vi "Get Shooter RPM.vi"(9 "Right Shooter Wheel":T1={"DeviceStatus"={"status"=FALSE, "code"=0, "source"=""}, "Type"=enum."PWM", "PWM"={"PWM Channel"=enum."Invalid", "DeadBand"={"Name"="", "maxPositivePwm"=0, "minPositivePwm"=0, "centerPwm"=0, "maxNegativePwm"=0, "minNegativePwm"=0, "angularRange"=0}}, "CAN"={"Device Number"=0, "Control Mode"=enum."Percent VBus", "Semaphore"=refnum, "Max Vout"=12.0, "TalonSRX Control Mode"=enum."Percent VBus"}, "Invert"=FALSE}, 11 "Left Shooter Wheel":T1={"DeviceStatus"={"status"=FALSE, "code"=0, "source"=""}, "Type"=enum."PWM", "PWM"={"PWM Channel"=enum."Invalid", "DeadBand"={"Name"="", "maxPositivePwm"=0, "minPositivePwm"=0, "centerPwm"=0, "maxNegativePwm"=0, "minNegativePwm"=0, "angularRange"=0}}, "CAN"={"Device Number"=0, "Control Mode"=enum."Percent VBus", "Semaphore"=refnum, "Max Vout"=12.0, "TalonSRX Control Mode"=enum."Percent VBus"}, "Invert"=FALSE}) -> (1 "Average RPM":dbl, 2 "Right RPM":dbl, 3 "Left RPM":dbl)   [LabVIEW 2015]
uses:
  <vilib>/Rock Robotics/WPI/MotorControl/WPI_MotorControlDeviceRef.ctl
  <vilib>/Rock Robotics/WPI/MotorControl/WPI_MotorControlType.ctl
  <vilib>/Rock Robotics/SystemInterfaces/DIO/FPGA_DIOPWMChannel.ctl
  <vilib>/Rock Robotics/WPI/PWM/WPI_PWMDeadband.ctl
  <vilib>/Rock Robotics/WPI/CAN/Jaguar/SubVIs/WPI_CANJaguar_ControlMode.ctl
  <vilib>/Rock Robotics/WPI/CAN/TalonSRX/WPI_CANTalonSRX_APIControlMode.ctl
  <vilib>/Rock Robotics/WPI/CAN/TalonSRX/WPI_CANTalonSRX_APIFeedbackSelect.ctl
  Robot Global Data.vi
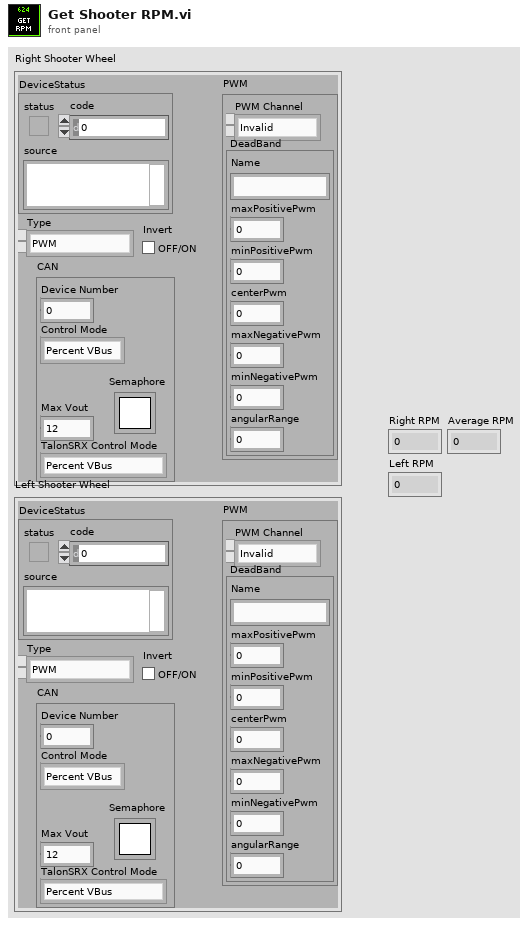
[diagram p1: front panel]
types:
  T1 = typedef "WPI_MotorControlDeviceRef.ctl" = cluster{"DeviceStatus":errorcluster, "Type":T2, "PWM":cluster{"PWM Channel":T3, "DeadBand":T4}, "CAN":cluster{"Device Number":u8, "Control Mode":T5, "Semaphore":T6, "Max Vout":dbl, "TalonSRX Control Mode":T7}, "Invert":bool}
  T2 = typedef "WPI_MotorControlType.ctl" = enum16{"PWM", "CAN", "CANTalonSRX"}
  T3 = typedef "FPGA_DIOPWMChannel.ctl" = enum8{"PWM 0", "PWM 1", "PWM 2", "PWM 3", "PWM 4", "PWM 5", "PWM 6", "PWM 7", "PWM 8", "PWM 9", "PWM MXP 0", "PWM MXP 1", "PWM MXP 2", "PWM MXP 3", "PWM MXP 4", "PWM MXP 5", "PWM MXP 6", "PWM MXP 7", "PWM MXP 8", "PWM MXP 9", "Invalid"}
  T4 = typedef "WPI_PWMDeadband.ctl" = cluster{"Name":string, "maxPositivePwm":i32, "minPositivePwm":i32, "centerPwm":i32, "maxNegativePwm":i32, "minNegativePwm":i32, "angularRange":u16}
  T5 = typedef "WPI_CANJaguar_ControlMode.ctl" = enum8{"Percent VBus", "Current", "Speed", "Position", "Voltage"}
  T6 = typedef "Semaphore RefNum" = refnum<k1>
  T7 = typedef "WPI_CANTalonSRX_APIControlMode.ctl" = enum8{"Percent VBus", "Speed", "Position", "Slave", "Unchanged / Invalid", "Voltage Compensation", "Current", "Motion Profile"}
  T8 = typedef "WPI_CANTalonSRX_APIFeedbackSelect.ctl" = enum16{"Digital Quadrature Encoder", "Analog Potentiometer", "Analog Encoder", "Count on Quad-A (Rising-Edge)", "Count on Quad-A (Falling-Edge)", "CTR Magnetic Enc (Absolute)", "CTR Magnetic Enc (Relative)", "Pulse Width"}
  T9 = typedef "Dashboard Control Data.ctl" = cluster{"Shooter Presets":T10, "Encoder Control":T12, "Steer PID output":cluster{"output high":dbl, "output low":dbl}, " Steer PID gains":cluster{"proportional gain (Kc)":dbl, "integral time (Ti, min)":dbl, "derivative time (Td, min)":dbl}, "Drivetrain Settings":T13, "Vision Packet":T14, "Dashboard Drivetrain Command":T15, "Info/Command Cluster":T17, "Ball Vision Packet":T18, "Intake Presets":T20, "Intake Encoder Control":T22, "Climb Presets":T23, "Ultrasonic Limit":dbl, "Roll Limit":dbl, "Pitch Limit":dbl, "Goal Output Range":cluster{"output high":dbl, "output low":dbl}}
  T10 = typedef "Shooter Presets.ctl" = cluster{"Batter Shot":T11, "Deep Middle Shot":T11, "Manual Shot":T11, "Left Ticks Per Rotation":dbl, "Right Ticks Per Rotation":dbl, "Low Bar Shot":T11, "Shooter RPM Tolerance":dbl, "IIR Filter Power":dbl, "Trigger Power":dbl, "Fire from Load Delay":i32, "Angle Pot M":dbl, "Angle Pot B":dbl, "Shooter Length":dbl, "String Pot Dist":dbl, "Angle PID gains":cluster{"proportional gain (Kc)":dbl, "integral time (Ti, min)":dbl, "derivative time (Td, min)":dbl}, "Angle Motor Output":cluster{"output high":dbl, "output low":dbl}, "Shooter Angle Tolerance":dbl, "Vision Shoot x^2":dbl, "Vision Shoot x":dbl, "Dist from Axis Cam to Pivot":dbl, "High Goal Center Height":dbl, "Feed Forward Max Accel":dbl, "Feed Forward Kv":dbl, "Backwards Trigger":dbl, "Shot Finish Delay (ms)":dbl, "Angle Max Current":dbl, "Angle Current Trip Time":dbl, "Shooter Intake Angle":dbl, "Vision Shoot c":dbl, "Reset?":bool, "Servo Release Delay":dbl, "Servo Idle Angle":i32, "Servo Hold Angle":i32, "Angle Pot x^2":dbl, "Angle Pot x":dbl, "Angle Pot c":dbl, "Ignore Angle?":bool}
  T11 = typedef "Shot Presets.ctl" = cluster{"Left Wheel RPM":dbl, "Right Wheel RPM":dbl, "Angle":dbl}
  T12 = typedef "Encoder Control.ctl" = cluster{"Right Tick Constant":dbl, "Left Tick Constant":dbl, "Reset?":bool, "Y Dist":cluster{"PID gains":cluster{"proportional gain (Kc)":dbl, "integral time (Ti, min)":dbl, "derivative time (Td, min)":dbl}}, "Y Stop Thresh":dbl, "Y Stop Speed":dbl}
  T13 = typedef "Drivetrain Settings.ctl" = cluster{"Gyro Tolerance":dbl, "Throttle Ramp (ms)":dbl, "Angular rate compensation":bool, "Throttle to Rate Scale":dbl, "Rate compensation gain":dbl, "Kv":dbl, "Ka":dbl, "Feed Forward P":dbl, "Feed Forward D":dbl, "Goal Vision PID gains":cluster{"proportional gain (Kc)":dbl, "integral time (Ti, min)":dbl, "derivative time (Td, min)":dbl}, "Goal Detection Window":dbl}
  T14 = typedef "Goal Vision Packet.ctl" = cluster{"Distance":dbl, "Center X":dbl, "Center Y":dbl, "Found Target?":bool}
  T15 = typedef "Dashboard Drivetrain Command.ctl" = cluster{"Drivetrain Vision":T16}
  T16 = typedef "Drivetrain Vision.ctl" = cluster{"Goal Window":dbl, "Ball Window":dbl}
  T17 = typedef "Ball Tracking Command Cluster.ctl" = cluster{"Distance to Ball":dbl, "Desired Angle":dbl, "Command":enum16{"Turn to Ball", "Turn to Angle", "Get Distance"}, "Pixels from Center":dbl}
  T18 = typedef "Ball Vision Packet.ctl" = cluster{"Ball Detected?":bool, "Distance to Ball":dbl, "Desired Angle":dbl, "Pixels from Center":dbl, "Tracking mode":T19}
  T19 = typedef "Tracking Mode.ctl" = enum16{"Turn to Ball", "Turn to Angle"}
  T20 = typedef "Intake Presets.ctl" = cluster{"Intake Speed":dbl, "Outake Speed":dbl, "Low Height":dbl, "Half Height":dbl, "Full Height":dbl, "Angle Speed":dbl, "Fast Angle":dbl, "Encoder Scale":dbl, "Load Height":dbl, "Output Range":T21, "Rotation Power Max/Min":dbl, "MaxCurrent":dbl, "Intake Trip Time":dbl, "Idle Height":dbl, "Max Height":dbl, "Reset Encoders?":bool, "PID gains":cluster{"proportional gain (Kc)":dbl, "integral time (Ti, min)":dbl, "derivative time (Td, min)":dbl}}
  T21 = typedef "Drivetrain Output Range.ctl" = cluster{"output high":dbl, "output low":dbl}
  T22 = typedef "IntakeEcoderControl.ctl" = cluster{"Arm Tick Constant":dbl, "Reset?":bool, "Y Dist":cluster{"PID gains":cluster{"proportional gain (Kc)":dbl, "integral time (Ti, min)":dbl, "derivative time (Td, min)":dbl}}, "Y Stop Thresh":dbl, "Y Stop Speed":dbl}
  T23 = typedef "Climb Presets.ctl" = cluster{"Pull Power":dbl, "Unpin Power":dbl, "Time to Hold":dbl}
  T24 = typedef "WPI_CANTalonSRX_GlobalStatus.ctl" = cluster{"Applied Throttle":dbl, "Module Enabled":bool, "CAN Error":errorcluster, "Closed Loop Error":dbl, "Forward Limit Switch Closed":bool, "Reverse Limit Switch Closed":bool, "Sensor Position":dbl, "Sensor Velocity":dbl, "Current":dbl, "Sticky Fault - Over Temp":bool, "Sticky Fault - Under Voltage":bool, "Sticky Fault - Forward Limit":bool, "Sticky Fault - Reverse Limit":bool, "Sticky Fault - Forward Soft Limit":bool, "Sticky Fault - Reverse Soft Limit":bool, "Brake is Enabled":bool, "Encoder Position":dbl, "Encoder Velocity":dbl, "Encoder Index Count":dbl, "Encoder A Pin State":bool, "Encoder B Pin State":bool, "Encoder Index Pin State":bool, "Analog In":dbl, "Analog In Velocity":dbl, "Temperature (C)":dbl, "Battery Voltage":dbl, "Control 5 Is Supported":bool, "Current Profile Slot Select":dbl, "Pos Div 8":bool, "Vel Div 4":bool, "Pulse Width Position":i32, "Pulse Width Velocity":i32, "Pulse Width Rise To Rise (us)":i32, "Pulse Width Rise To Fall (us)":i32, "Mot Prof Active Is Under Run":bool, "Mot Prof Active Has Under Run":bool, "Mot Prof Active Is Last":bool, "Mot Prof Active Velocity Only":bool, "Mot Prof Active Is Valid":bool, "Mot Prof Buffer Is Full":bool, "Mot Prof Active Profile Slot Select":i32, "Mot Prof NextID":i32, "Mot Prof Count":i32, "Mot Prof Active Velocity":dbl, "Mot Prof Active Position":dbl, "Mot Prof Output Enable":i32}
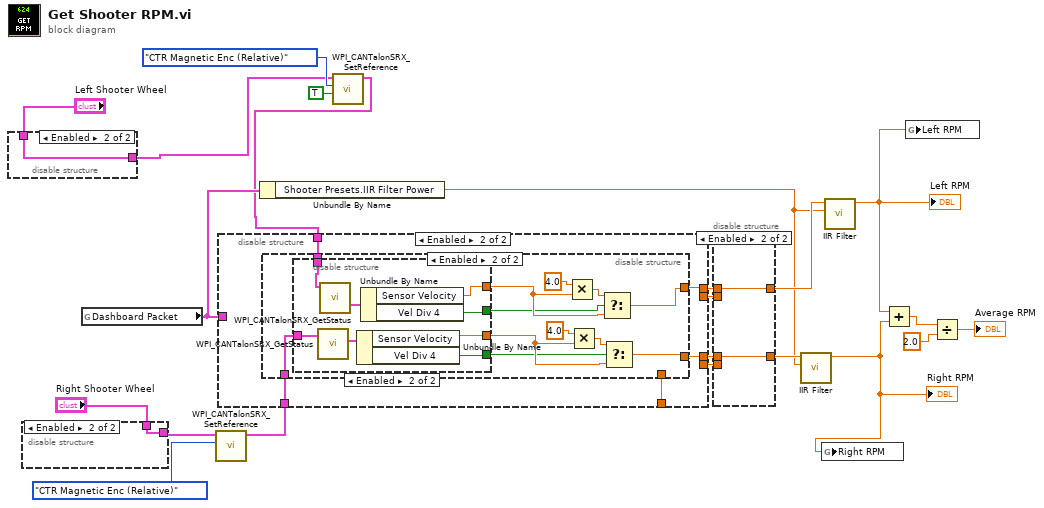
[diagram p0: block diagram]
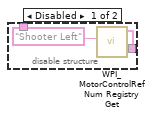
[diagram p2: hidden frame]
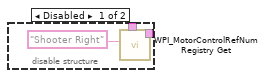
[diagram p3: hidden frame]
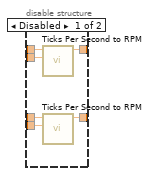
[diagram p4: hidden frame]
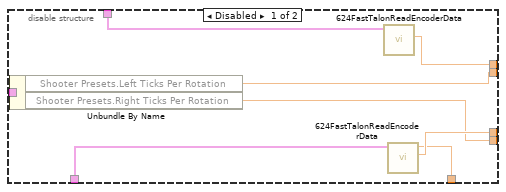
[diagram p5: hidden frame]
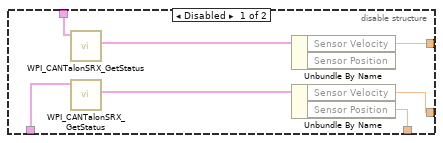
[diagram p6: hidden frame]
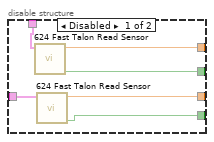
[diagram p7: hidden frame]
diagram:
  n1 = disable-structure shown="Enabled" {
    disable-tunnel: [w23 w25] -> w3
    disable-tunnel: "Left Shooter Wheel" -> [_ w25]
    frame Disabled {
      n2 = call <vilib>:"WPI_MotorControlRefNum Registry Get.vi"("refnum name"="Shooter Left") -> ("MotorControlDevRef"=w23:T1)  [unwired: 9 in, 1 out]
    }
    frame Enabled {
    }
  }
  n3 = disable-structure shown="Enabled" {
    disable-tunnel: [w26 w28] -> w7
    disable-tunnel: "Right Shooter Wheel" -> [_ w28]
    frame Disabled {
      n4 = call <vilib>:"WPI_MotorControlRefNum Registry Get.vi"("refnum name"="Shooter Right") -> ("MotorControlDevRef"=w26:T1)  [unwired: 9 in, 1 out]
    }
    frame Enabled {
    }
  }
  n5 = global read "Robot Global Data.vi" "Dashboard Packet"() -> (w15:T9)
  n6 = call <vilib>:"WPI_CANTalonSRX_SetReference.vi"("Feedback Reference"=WPI_CANTalonSRX_APIFeedbackSelect."CTR Magnetic Enc (Relative)", "CAN Talon SRX Ref"=w7) -> ("CAN Talon SRX Ref"=w5:T1)  [unwired: 8 in, 1 out]
  n7 = Unbundle By Name(w15) -> ("Shooter Presets.IIR Filter Power"=w12:dbl)
  n8 = call <vilib>:"WPI_CANTalonSRX_SetReference.vi"("Reverse Feedback Sensor"=TRUE, "Feedback Reference"=WPI_CANTalonSRX_APIFeedbackSelect."CTR Magnetic Enc (Relative)", "CAN Talon SRX Ref"=w3) -> ("CAN Talon SRX Ref"=w2:T1)  [unwired: 7 in, 1 out]
  n9 = disable-structure shown="Enabled" {
    disable-tunnel: [w36 w37] -> w22
    disable-tunnel: [w35 _] -> w21
    disable-tunnel: [w34 w40] -> w20
    disable-tunnel: [w33 _] -> w19
    disable-tunnel: w15 -> [w32 _]
    disable-tunnel: [w31 w39] -> _
    disable-tunnel: w2 -> [w30 w38]
    disable-tunnel: w5 -> [w29 w41]
    frame Disabled {
      n10 = Unbundle By Name(w32) -> ("Shooter Presets.Left Ticks Per Rotation"=w35:dbl, "Shooter Presets.Right Ticks Per Rotation"=w33:dbl)
      n11 = call "624FastTalonReadEncoderData.vi"("CAN Talon SRX Ref"=w30) -> ("Sensor RPM"=w36:dbl)  [unwired: 9 in, 1 out]
      n12 = call "624FastTalonReadEncoderData.vi"("CAN Talon SRX Ref"=w29) -> ("Sensor RPM"=w34:dbl, "Sensor Position"=w31:dbl)  [unwired: 9 in]
    }
    frame Enabled {
      n13 = disable-structure shown="Enabled" {
        disable-tunnel: w41 -> [w48 w60]
        disable-tunnel: [w46 w56] -> w40
        disable-tunnel: [w45 _] -> w39
        disable-tunnel: w38 -> [w43 w51]
        disable-tunnel: [w42 w50] -> w37
        frame Disabled {
          n14 = call <vilib>:"WPI_CANTalonSRX_GetStatus.vi"("CAN Talon SRX Ref"=w43) -> ("Talon SRX Status"=w44:T24)  [unwired: 8 in, 2 out]
          n15 = call <vilib>:"WPI_CANTalonSRX_GetStatus.vi"("CAN Talon SRX Ref"=w48) -> ("Talon SRX Status"=w47:T24)  [unwired: 8 in, 2 out]
          n16 = Unbundle By Name(w44) -> ("Sensor Velocity"=w42:dbl)  [unwired: 1 out]
          n17 = Unbundle By Name(w47) -> ("Sensor Velocity"=w46:dbl, "Sensor Position"=w45:dbl)
        }
        frame Enabled {
          n18 = disable-structure shown="Enabled" {
            disable-tunnel: w60 -> [w66 w74]
            disable-tunnel: [w65 w69] -> w59
            disable-tunnel: [w64 w70] -> w53
            disable-tunnel: [w63 w67] -> w52
            disable-tunnel: w51 -> [w62 w73]
            disable-tunnel: [w61 w68] -> w49
            frame Disabled {
              n19 = call "624 Fast Talon Read Sensor.vi"("MotorControlDevRef"=w62) -> ("V Div By 4"=w63:bool, "Sensor RPM"=w64:dbl)  [unwired: 7 in, 2 out]
              n20 = call "624 Fast Talon Read Sensor.vi"("MotorControlDevRef"=w66) -> ("V Div By 4"=w61:bool, "Sensor RPM"=w65:dbl)  [unwired: 7 in, 2 out]
            }
            frame Enabled {
              n21 = call <vilib>:"WPI_CANTalonSRX_GetStatus.vi"("CAN Talon SRX Ref"=w74) -> ("Talon SRX Status"=w71:T24)  [unwired: 8 in, 2 out]
              n22 = call <vilib>:"WPI_CANTalonSRX_GetStatus.vi"("CAN Talon SRX Ref"=w73) -> ("Talon SRX Status"=w72:T24)  [unwired: 8 in, 2 out]
              n23 = Unbundle By Name(w71) -> ("Sensor Velocity"=w69:dbl, "Vel Div 4"=w68:bool)
              n24 = Unbundle By Name(w72) -> ("Sensor Velocity"=w70:dbl, "Vel Div 4"=w67:bool)
            }
          }
          n25 = Multiply(x=4.0, y=w53) -> (x*y=w55:dbl)
          n26 = Multiply(x=4.0, y=w59) -> (x*y=w57:dbl)
          n27 = Select(t=w55, s=w52, f=w53) -> (s? t:f=w50:dbl)
          n28 = Select(t=w57, s=w49, f=w59) -> (s? t:f=w56:dbl)
        }
      }
    }
  }
  n29 = disable-structure shown="Enabled" {
    disable-tunnel: w22 -> [w80 w82]
    disable-tunnel: w21 -> [w79 _]
    disable-tunnel: w20 -> [w78 w81]
    disable-tunnel: w19 -> [w77 _]
    disable-tunnel: [w76 w82] -> w14
    disable-tunnel: [w75 w81] -> w13
    frame Disabled {
      n30 = call "Ticks Per Second to RPM.vi"("Ticks per Rotation"=w79, "Ticks Per Second"=w80) -> ("RPM"=w76:dbl)  [unwired: 9 in]
      n31 = call "Ticks Per Second to RPM.vi"("Ticks per Rotation"=w77, "Ticks Per Second"=w78) -> ("RPM"=w75:dbl)  [unwired: 9 in]
    }
    frame Enabled {
    }
  }
  n32 = call "IIR Filter.vi"("Filter Power"=w12, "Value"=w13) -> ("Filtered Value"=w8:dbl)  [unwired: 9 in]
  "Right RPM" <- w8
  n33 = global write "Robot Global Data.vi" "Right RPM"(w8) -> ()
  n34 = call "IIR Filter.vi"("Filter Power"=w12, "Value"=w14) -> ("Filtered Value"=w9:dbl)  [unwired: 9 in]
  "Left RPM" <- w9
  n35 = Add(x=w9, y=w8) -> (x+y=w18:dbl)
  n36 = global write "Robot Global Data.vi" "Left RPM"(w9) -> ()
  n37 = Divide(x=w18, y=2.0) -> (x/y=→"Average RPM":dbl)
